vi "Fetch Multi Eval Meas SEM Trace Area Results.vi"(6 "Area (1)":T2=1, 7 "Offset Frequency (Positive)":T1=1 items=["Negative", "Positive"], 8 "error in (no error)":errorcluster, 9 "Result Type (Current)":i32(ring) items=["Current"=0, "Average"=1, "Maximum"=4], 10 "Instance (1)":T3=1, 11 "VISA resource name":refnum<visa-resource-name>) -> (0 "error out":errorcluster, 1 "Results":dbl[](array[numeric]) format="%^.3e", 2 "Reliability":i32, 3 "VISA resource name out":refnum<visa-resource-name>, 4 "Resolution BW":i32)   [LabVIEW 2020, in "Rohde&Schwarz CMWXP NR FR1 Measurement.lvlib"]
doc: "Returns the measured power values for a single spectrum emission mask area with enabled limit check.\n\nThe results of the current, average and maximum traces can be retrieved. The area is located below (negative) or above (positive) the carrier center frequency.\n\nAttributes:\nRSCMWXPNRFR1M_ATTR_FETCH_MULTI_EVAL_MEAS_SEM_AREA_POSITIVE_CURRENT_RESULTS\nRSCMWXPNRFR1M_ATTR_FETCH_MULTI_EVAL_MEAS_SEM_AREA_POSITIVE_AVERAGE_RESULTS\nRSCMWXPNRFR1M_ATTR_FETCH_MULTI_EVAL_MEAS_SEM_AREA_POSITIVE_MAXIMUM_RESULTS\nRSCMWXPNRFR1M_ATTR_FETCH_MULTI_EVAL_MEAS_SEM_AREA_NEGATIVE_CURRENT_RESULTS\nRSCMWXPNRFR1M_ATTR_FETCH_MULTI_EVAL_MEAS_SEM_AREA_NEGATIVE_AVERAGE_RESULTS\nRSCMWXPNRFR1M_ATTR_FETCH_MULTI_EVAL_MEAS_SEM_AREA_NEGATIVE_MAXIMUM_RESULTS\n\nRemote-control commands:\nFETCh:NRSub:MEAS<i>:MEValuation:TRACe:SEMask:AREA<area>:POSitive:CURRent?\nFETCh:NRSub:MEAS<i>:MEValuation:TRACe:SEMask:AREA<area>:POSitive:AVERage?\nFETCh:NRSub:MEAS<i>:MEValuation:TRACe:SEMask:AREA<area>:POSitive:MAXimum?\nFETCh:NRSub:MEAS<i>:MEValuation:TRACe:SEMask:AREA<area>:NEGative:CURRent?\nFETCh:NRSub:MEAS<i>:MEValuation:TRACe:SEMask:AREA<area>:NEGative:AVERage?\nFETCh:NRSub:MEAS<i>:MEValuation:TRACe:SEMask:AREA<area>:NEGative:MAXimum?"
uses:
  <instrlib>/Rohde&Schwarz CMWXP NR FR1 Measurement/Rohde&Schwarz CMWXP NR FR1 Measurement.lvlib
  <instrlib>/Rohde&Schwarz CMWXP NR FR1 Measurement/Private/_Instance.ctl
  <instrlib>/Rohde&Schwarz CMWXP NR FR1 Measurement/Private/_Area.ctl
  <instrlib>/Rohde&Schwarz CMWXP NR FR1 Measurement/Private/_Offset Frequency.ctl
  <instrlib>/Rohde&Schwarz CMWXP NR FR1 Measurement/Private/rsidr_core.llb/rsidr_core.lvlib
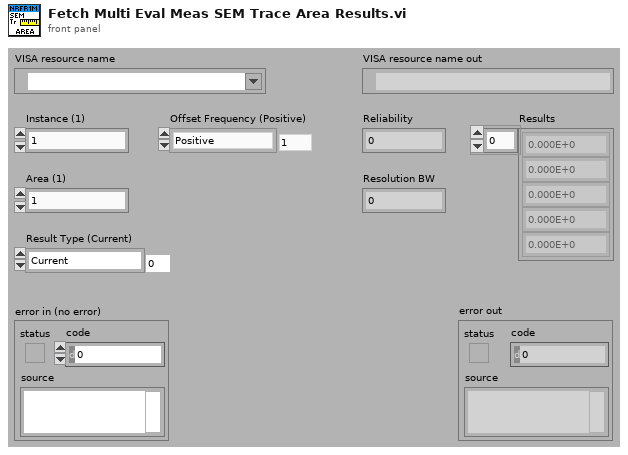
[diagram p1: front panel]
types:
  T1 = typedef "Rohde&Schwarz CMWXP NR FR1 Measurement.lvlib/_Offset Frequency.ctl" = i32
  T2 = typedef "Rohde&Schwarz CMWXP NR FR1 Measurement.lvlib/_Area.ctl" = i32
  T3 = typedef "Rohde&Schwarz CMWXP NR FR1 Measurement.lvlib/_Instance.ctl" = i32
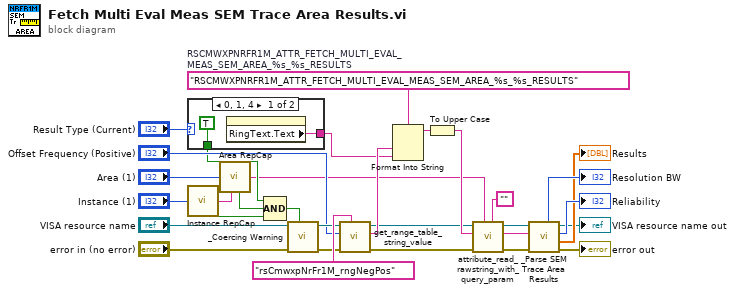
[diagram p0: block diagram]
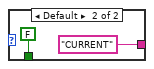
[diagram p2: hidden frame]
diagram:
  w19 = "RSCMWXPNRFR1M_ATTR_FETCH_MULTI_EVAL_MEAS_SEM_AREA_%s_%s_RESULTS"  # RSCMWXPNRFR1M_ATTR_FETCH_MULTI_EVAL_MEAS_SEM_AREA_%s_%s_RESULTS
  n1 = case shown="0, 1, 4" "Result Type (Current)" {
    tunnel: [w32 "CURRENT"] -> w14
    tunnel: [TRUE FALSE] -> w16
    frame 0, 1, 4 {
      n2 = property on="Result Type (Current)" class="Ring (strict)"() -> ("RingText.Text"=w32:string)  [unwired: 2 in, 2 out]
    }
    frame Default {
    }
  }
  n3 = call <instrlib>:"Instance RepCap.vi"("Instance In"="Instance (1)") -> ("In Range?"=w28:bool, "RepCap Identifier Out"=w27:string)  [unwired: 1 in]
  n4 = call <instrlib>:"Area RepCap.vi"("SEM Area In"="Area (1)", "RepCap String In (\"\")"=w27) -> ("In Range?"=w26:bool, "RepCap Identifier Out"=w12:string)
  n5 = Compound Arithmetic op=AND(w16, w26, w28) -> (w29:bool)
  n6 = call <instrlib>:"_Coercing Warning.vi"("In Range?"=w29, "error in (no error)"="error in (no error)", "VISA resource name"="VISA resource name") -> ("error out"=w21:errorcluster, "VISA resource name out"=w22:refnum<visa-resource-name>)  [unwired: 7 in]
  n7 = call <instrlib>:"get_range_table_string_value.vi"("Range Table ID in"="rsCmwxpNrFr1M_rngNegPos", "error in"=w21, "I32 input"="Offset Frequency (Positive)", "VISA resource name"=w22) -> ("error out"=w9:errorcluster, "String Value out"=w15:string, "VISA resource name out"=w10:refnum<visa-resource-name>)  [unwired: 5 in]
  n8 = Format Into String(format string=w19, w15, w14) -> (resulting string=w18:string)  [unwired: 2 in, 1 out]
  n9 = To Upper Case(1:w18) -> (0:w13:string)
  n10 = call <instrlib>:"attribute_read_rawstring_with_query_param.vi"("Query Parameter (None)"="", "Repeated Capability"=w12, "error in"=w9, "Attribute ID"=w13, "VISA resource name"=w10) -> ("error out"=w6:errorcluster, "Raw String out"=w7:string, "VISA resource name out"=w8:refnum<visa-resource-name>)  [unwired: 4 in]
  n11 = call <instrlib>:"_Parse SEM Trace Area Results.vi"("error in (no error)"=w6, "Input String"=w7, "VISA resource name"=w8) -> ("error out"=→"error out":errorcluster, "Results"=→"Results":dbl[], "Reliability"=→"Reliability":i32, "VISA resource name out"=→"VISA resource name out":refnum<visa-resource-name>, "Resolution BW"=→"Resolution BW":i32)  [unwired: 4 in]
